vi "Draw Picture.vi"(10 "picture in":picture, 11 "Flying Saucer in":refnum<class "Flying Saucer.lvclass">) -> (2 "picture out":picture)   [LabVIEW 2024, in "Flying Saucer.lvclass"]
doc: "MIT Licence\nCopyright (c) 2024 David Grollier"
uses:
  Flying Saucer.lvclass
  Game Board Component.lvclass/Game Board Component.ctl
  Movable.lvclass/Movable.ctl
  Flying Saucer.lvclass/Flying Saucer.ctl
  Movable.lvclass
  Game Board Component.lvclass
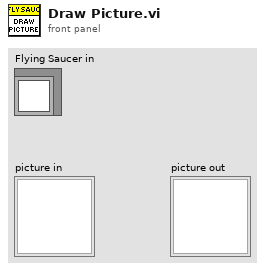
[diagram p1: front panel]
types:
  T1 = typedef "Velocity.ctl" = cluster{"Vx":dbl, "Vy":dbl}
  T2 = typedef "Coordinates.ctl" = cluster{"x":dbl, "y":dbl}
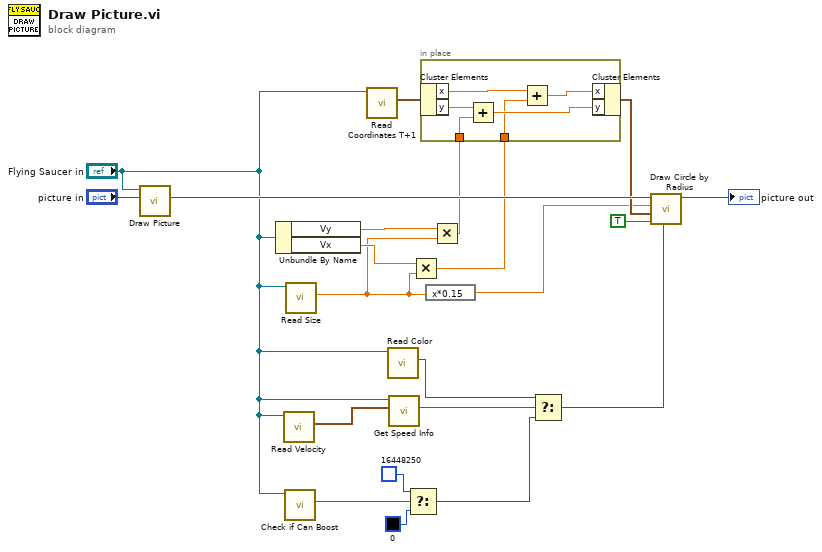
[diagram p0: block diagram]
diagram:
  n1 = call-parent "Draw Picture.vi"("picture in"="picture in", "Movable in"="Flying Saucer in") -> ("picture out"=w20:picture)  [unwired: 9 in]
  n2 = Unbundle By Name("Flying Saucer in") -> ("Vy"=w14:dbl, "Vx"=w13:dbl)
  n3 = call-dynamic "Read Velocity.vi"("Movable in"="Flying Saucer in") -> ("Velocity"=w12:T1)  [unwired: 10 in]
  n4 = call "Check if Can Boost.vi"("Flying Saucer in"="Flying Saucer in") -> ("Can Boost?"=w9:bool)  [unwired: 10 in]
  n5 = call "Read Size.vi"("Movable in"="Flying Saucer in") -> ("Size"=w2:dbl)  [unwired: 10 in]
  n6 = call "Read Coordinates T+1.vi"("Movable in"="Flying Saucer in") -> ("Coordinates"=w3:T2)  [unwired: 10 in]
  n7 = call "Read Color.vi"("Game Board Component in"="Flying Saucer in") -> ("color"=w6:u32)  [unwired: 10 in]
  n8 = call "Get Speed Info.vi"("Velocity in"=w12, "Movable in"="Flying Saucer in") -> ("Max speed?"=w8:bool)  [unwired: 8 in, 1 out]
  n9 = Select(t=u32 16448250 ("color(black)"), s=w9, f=u32 0 ("color(black)")) -> (s? t:f=w7:u32)
  n10 = Multiply(x=w13, y=w2) -> (x*y=w16:dbl)
  n11 = expression code="x*0.15"(w2) -> (w17:dbl)
  n12 = Multiply(x=w14, y=w2) -> (x*y=w15:dbl)
  n13 = in-place {
    in-place-border: w16 -> [w23]
    in-place-border: w15 -> [w22]
    n14 = in-place-cluster #1(w3) -> ("x"=w27:dbl, "y"=w25:dbl)
    n15 = Add(x=w25, y=w22) -> (x+y=w24:dbl)
    n16 = Add(x=w27, y=w23) -> (x+y=w26:dbl)
    n17 = in-place-cluster #1("x"=w26, "y"=w24) -> (w18:T2)
  }
  n18 = Select(t=w6, s=w8, f=w7) -> (s? t:f=w5:u32)
  n19 = call <vilib>:"Draw Circle by Radius.vi"("color(black)"=w5, "fill?(F)"=TRUE, "pixel center"=w18, "radius"=w17, "picture"=w20) -> ("new picture"=→"picture out":picture)  [unwired: 6 in]
